vi "array1.vi"() -> ()   [LabVIEW 2020]
panel:
  out "Numeric 3":i32
  out "Array":i32[](array[numeric])
  out "Numeric 2":i32
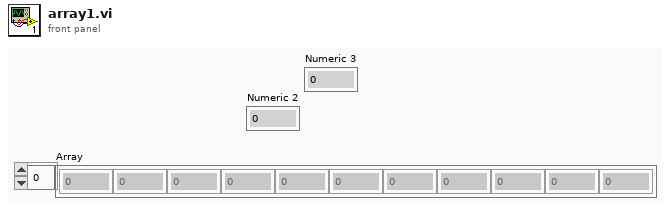
[diagram p1: front panel]
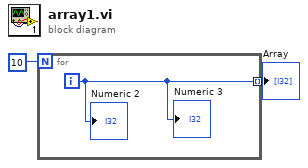
[diagram p0: block diagram]
diagram:
  n1 = for {
    N: 10 -> [_]
    tunnel: [w3] -> w1 mode=indexing
    i -> [w3]
    "Numeric 2" <- w3
    "Numeric 3" <- w3
  }
  "Array" <- w1
